vi "Drive Controller.vi"(8 "error in":errorcluster) -> ()   [LabVIEW 2017]
doc: "This VI executes continuously carrying out the current operation and responding to updates or new operation requests. It will often contain the timing or control code that is difficult to place directly in TeleOp. This VI generally opens all sensors and motors and isolates the rest of the robot code from knowing implementation details of how the operations are carried out."
uses:
  <vilib>/Rock Robotics/WPI/Framework/Completion Status.ctl
  Drive Setpoints.ctl
  Drive Operations.ctl
  <vilib>/Rock Robotics/WPI/SafetyOutput/WPI_SafetyOutputConfigMenu.ctl
  <vilib>/Rock Robotics/SystemInterfaces/DIO/FPGA_DIOChannel.ctl
  <vilib>/Rock Robotics/SystemInterfaces/DIO/FPGA_DIOPWMChannel.ctl
  <vilib>/Rock Robotics/WPI/Counter/WPI_CounterDigitalInputToDigitalSource.vi
  Framework/Robot Global Data.vi
  <vilib>/Rock Robotics/WPI/ThirdParty/Phoenix-LabVIEW/Pigeon IMU/CTRE_PigeonIMU_Open_TalonSRX.vi
  <vilib>/Rock Robotics/Network Tables/NT Write Number.vi
  <vilib>/Rock Robotics/WPI/RobotDrive/WPI_RobotDriveOpen4MotorWithSPARK.vi
  Support Code/Global Constants.vi
  <vilib>/Rock Robotics/Network Tables/NT Write Numeric Array.vi
panel:
  in  "PID Turn":T1={"proportional gain (Kc)"=0.015, "integral time (Ti, min)"=0.0, "derivative time (Td, min)"=0.0}
  in  "Sensitivity":dbl=0.2 format="%#_13g"
  out "Encoders":cluster{"Distance":dbl, "Distance":dbl}(graph)
  out "Left Encoder":dbl=-1185.6884765625
  out "Right Encoder":dbl=-1185.6884765625
  out "gyro":dbl=106.72
  out "Gyro":dbl(graph)=85.48
  in  "Interactive Values":T2={"Operation"=enum."Auto Turn", "Left Setpoint"=0.0, "Right Setpoint"=0.0, "Duration"=0.0, "Distance"=0.0, "Target Angle"=90.0, "Speed"=0.0}
  in  "Buttons":cluster{"Execute Cmd":bool, "Abort Cmd":bool}
  out "Command Timing":cluster{"Start Time (ms)":u32, "Iterations":i32}={"Start Time (ms)"=2214017, "Iterations"=0}
  out "Status":T4
  out "Setpoints":T5(graph)
  out "Current\nCmd":string="Started at  17:19:58.001\nDefault: Reserve,  L 0.0, R 0.0, D 0.000000, Dist 0.0, A 0.0, S 0.000000"
  # "Interactive Command: You may fill in the settings for a command\nand schedule it with the Execute button. You can observe and abort\nany command while fine tuning the code for the controller."
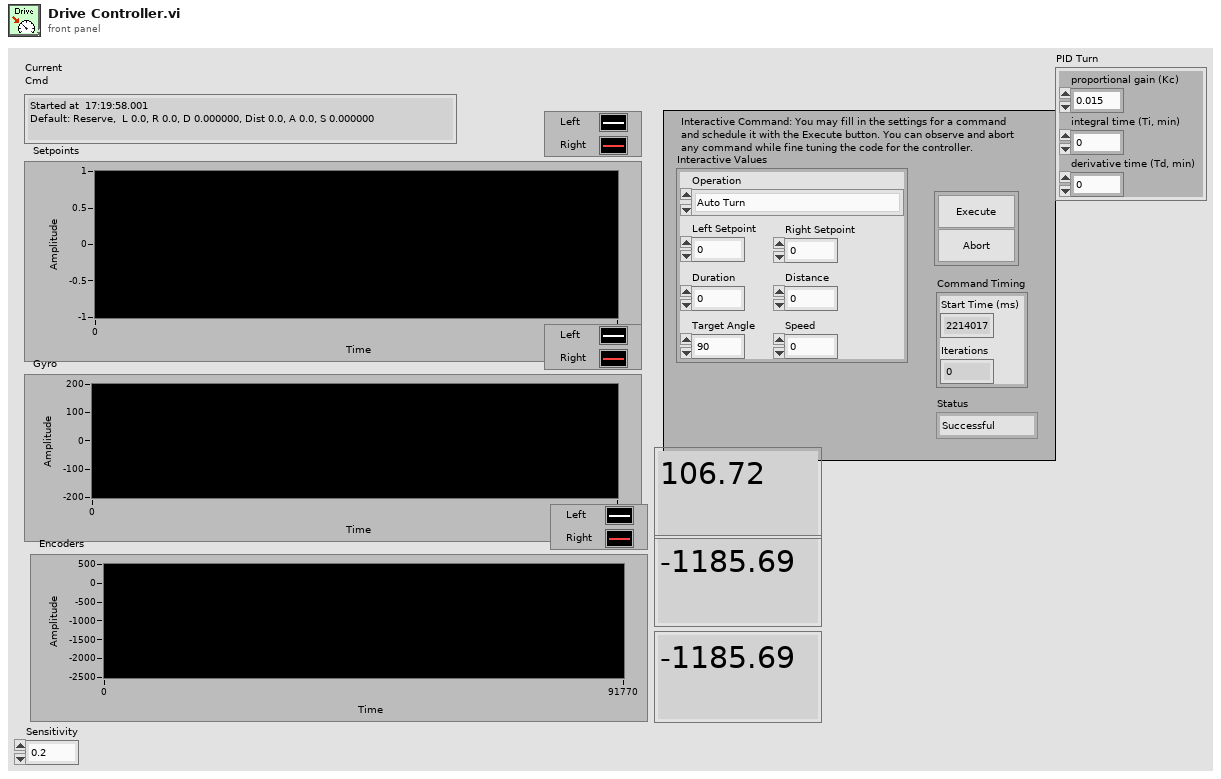
[diagram p1: front panel]
types:
  T1 = cluster{"proportional gain (Kc)":dbl, "integral time (Ti, min)":dbl, "derivative time (Td, min)":dbl}
  T2 = typedef "Drive Setpoints.ctl" = cluster{"Operation":T3, "Left Setpoint":dbl, "Right Setpoint":dbl, "Duration":dbl, "Distance":dbl, "Target Angle":dbl, "Speed":dbl}
  T3 = typedef "Drive Operations.ctl" = enum16{"Reserve", "Read Current", "Immediate", "Drive for Time", "Drive for Distance", "Drive PID", "Auto Turn", "Reset Encoders", "Reset Gyro"}
  T4 = typedef "Completion Status.ctl" = enum16{"Successful", "Aborted", "Incomplete"}
  T5 = cluster{"Left Setpoint":dbl, "Right Setpoint":dbl}
  T6 = typedef "FPGA_DIOPWMChannel.ctl" = enum8{"PWM 0", "PWM 1", "PWM 2", "PWM 3", "PWM 4", "PWM 5", "PWM 6", "PWM 7", "PWM 8", "PWM 9", "PWM MXP 0", "PWM MXP 1", "PWM MXP 2", "PWM MXP 3", "PWM MXP 4", "PWM MXP 5", "PWM MXP 6", "PWM MXP 7", "PWM MXP 8", "PWM MXP 9", "Invalid"}
  T7 = typedef "FPGA_DIOChannel.ctl" = enum8{"DIO 0", "DIO 1", "DIO 2", "DIO 3", "DIO 4", "DIO 5", "DIO 6", "DIO 7", "DIO 8", "DIO 9", "DIO MXP 0", "DIO MXP 1", "DIO MXP 2", "DIO MXP 3", "DIO MXP 4", "DIO MXP 5", "DIO MXP 6", "DIO MXP 7", "DIO MXP 8", "DIO MXP 9", "DIO MXP 10", "DIO MXP 11", "DIO MXP 12", "DIO MXP 13", "DIO MXP 14", "DIO MXP 15", "SPI Port CS1", "SPI Port CS2", "SPI Port CS3", "SPI Port MISO", "SPI Port MOSI", "Invalid"}
  T8 = typedef "WPI_SafetyOutputConfigMenu.ctl" = enum16{"Enable", "Disable"}
  T9 = typedef "WPI_MotorControlDeviceRef.ctl" = cluster{"DeviceStatus":errorcluster, "Type":T10, "PWM":cluster{"PWM Channel":T6, "DeadBand":T11}, "CAN":cluster{"Device Number":u8, "SetOutput VI Ref":variant, "GetOutput VI Ref":variant, "Enable VI Ref":variant, "Disable VI Ref":variant, "Data":variant}, "Invert":bool, "DIO PWM":cluster{"PWM \"Enable\" Channel":T6, "DIOChannel":T7, "PWM Rate":dbl}}
  T10 = typedef "WPI_MotorControlType.ctl" = enum16{"PWM", "CAN", "DIO PWM"}
  T11 = typedef "WPI_PWMDeadband.ctl" = cluster{"Name":string, "maxPositivePwm":i32, "minPositivePwm":i32, "centerPwm":i32, "maxNegativePwm":i32, "minNegativePwm":i32, "angularRange":u16}
  T12 = typedef "CTRE_PigeonIMU_DeviceRef.ctl" = cluster{"DeviceStatus":errorcluster, "Device Number":u8, "Type":T13, "Device ID":u32, "Handle":u64, "UsageFrame":u32, "Library Path":path}
  T13 = typedef "CTRE_PigeonIMU_ConnectionType.ctl" = u32
  T14 = typedef "WPI_DigitalInputDevRef.ctl" = cluster{"DevStatus":errorcluster, "DIO Channel":T7}
  T15 = typedef "WPI_RobotDriveDevRef.ctl" = cluster{"DevStatus":errorcluster, "Motors[]":T9[], "Square Inputs":bool, "Max Output":dbl}
  T16 = typedef "FPGA_CounterEncoderSourceConvertionLVSourceType.ctl" = cluster{"DevStatus":errorcluster, "AnalogTriggerMode?":bool, "DigitalMode":cluster{"DIO Channel":T17}, "AnalogTriggerMode":cluster{"AnalogTriggerIndex":T18, "OutputType":T19}}
  T17 = typedef "FPGA_DIODigitalSourceChannel.ctl" = enum8{"DIO 0", "DIO 1", "DIO 2", "DIO 3", "DIO 4", "DIO 5", "DIO 6", "DIO 7", "DIO 8", "DIO 9", "DIO MXP 0", "DIO MXP 1", "DIO MXP 2", "DIO MXP 3", "DIO MXP 4", "DIO MXP 5", "DIO MXP 6", "DIO MXP 7", "DIO MXP 8", "DIO MXP 9", "DIO MXP 10", "DIO MXP 11", "DIO MXP 12", "DIO MXP 13", "DIO MXP 14", "DIO MXP 15", "Disabled"}
  T18 = typedef "FPGA_AnalogTriggerIndex.ctl" = enum8{"Trig 0", "Trig 1", "Trig 2", "Trig 3", "Trig 4", "Trig 5", "Trig 6", "Trig 7", "Invalid"}
  T19 = typedef "FPGA_AnalogTriggerOutType.ctl" = enum16{"InWindow", "TriggerState", "Rising", "Falling"}
  T20 = typedef "WPI_EncoderDevRef.ctl" = cluster{"DevStatus":errorcluster, "EncoderIndex":T21, "CounterIndex":T22, "DistancePerCount":dbl, "Decoding Type":T23}
  T21 = typedef "FPGA_EncoderIdx.ctl" = enum8{"Enc 0", "Enc 1", "Enc 2", "Enc 3", "Enc 4", "Enc 5", "Enc 6", "Enc 7", "Invalid"}
  T22 = typedef "FPGA_CounterCtrSystemIndex.ctl" = enum8{"Ctr 0", "Ctr 1", "Ctr 2", "Ctr 3", "Ctr 4", "Ctr 5", "Ctr 6", "Ctr 7", "Invalid"}
  T23 = typedef "WPI_EncoderType.ctl" = enum16{"1x", "2x", "4x"}
  T24 = typedef "Command Status Info.ctl" = cluster{"Name":string, "Status":T4, "notifier out":T25}
  T25 = typedef "Completion Notifier.ctl" = refnum<notifier>
  T26 = cluster{"SubSystem Data":T2, cluster{"Start Time (ms)":u32, "Iterations":i32}, cluster{"Command Info":T24, "Description":string, "Default Command":T2, "queue out":refnum<queue>, "Subsystem Name":string}}
  T27 = cluster{"SubSystem Data":T2, cluster{"Start Time (ms)":u32, "Iterations":i32}, "Default Command Arguments":cluster{"Command Info":T24, "Description":string, "Default Command":T2, "queue out":refnum<queue>, "Subsystem Name":string}}
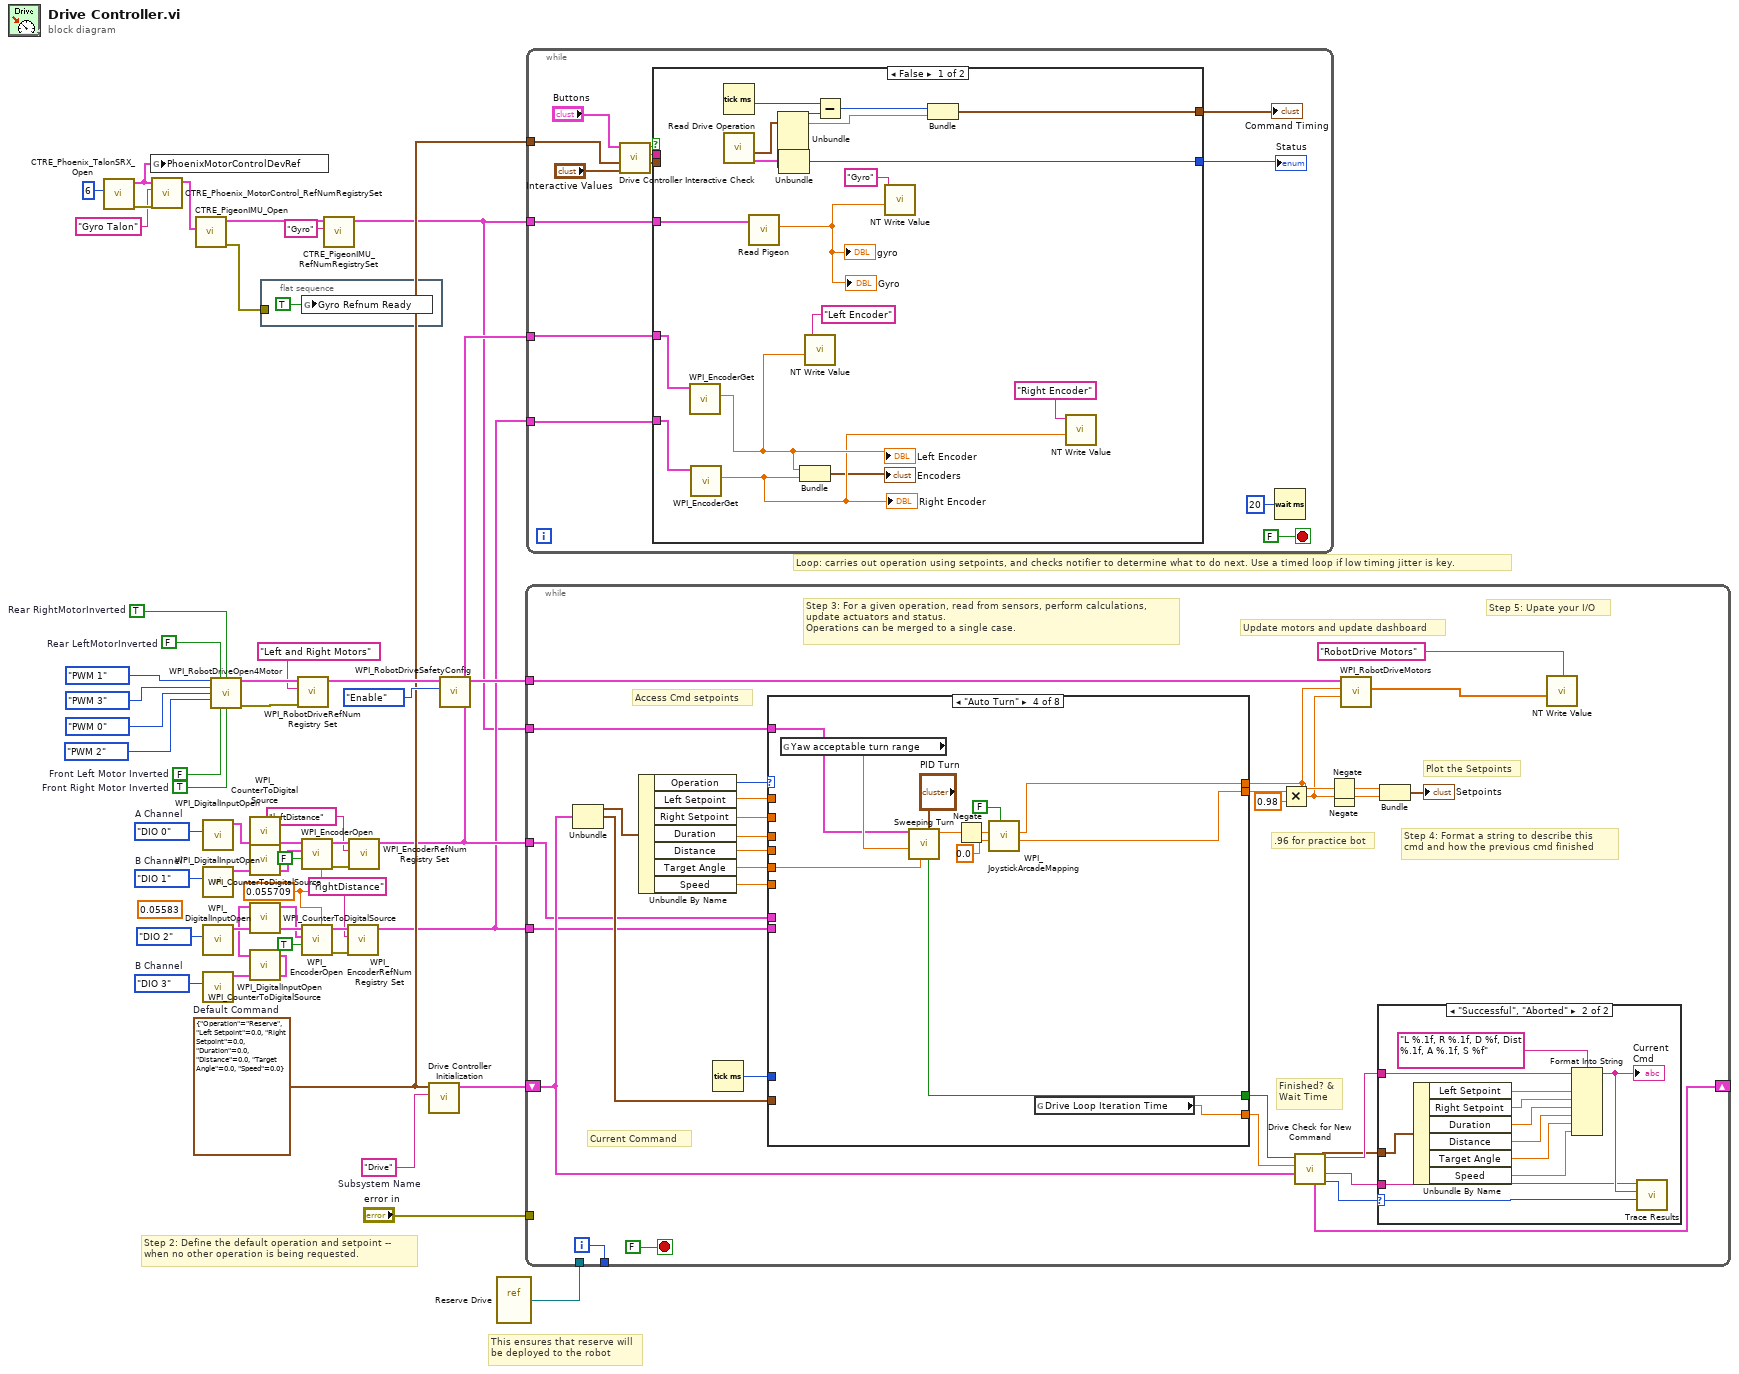
[diagram p0: block diagram]
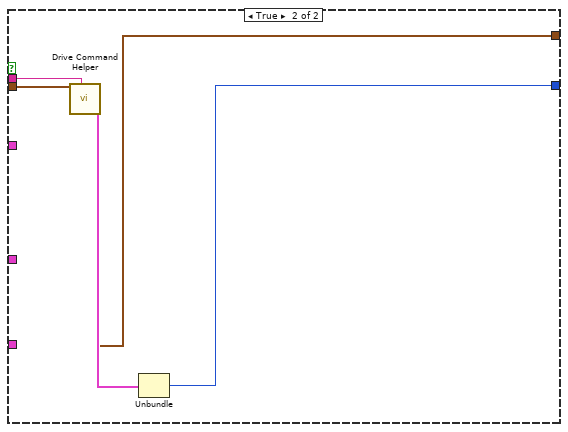
[diagram p2: hidden frame]
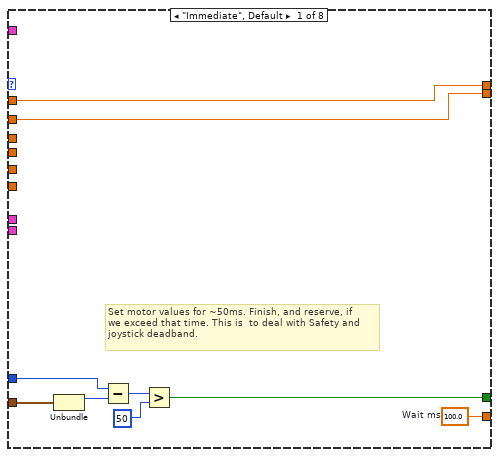
[diagram p4: hidden frame]
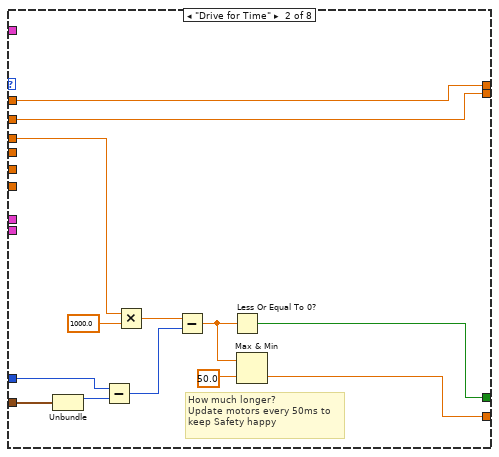
[diagram p5: hidden frame]
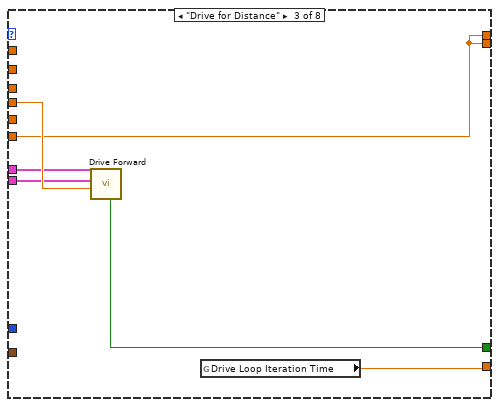
[diagram p6: hidden frame]
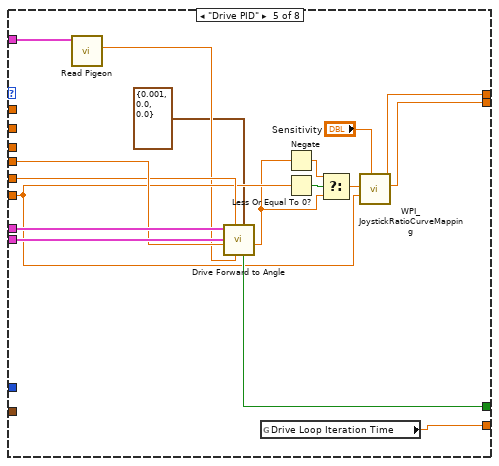
[diagram p7: hidden frame]
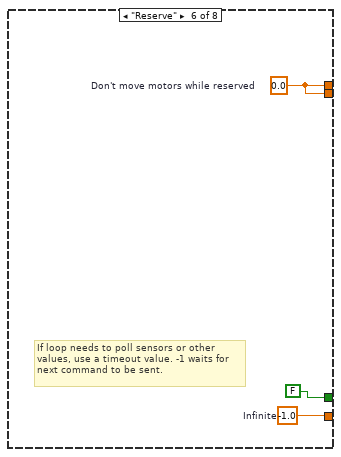
[diagram p8: hidden frame]
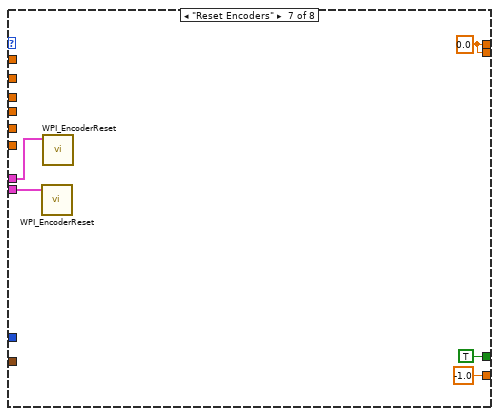
[diagram p9: hidden frame]
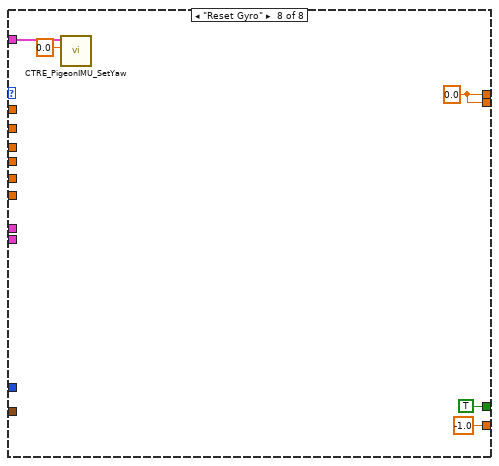
[diagram p10: hidden frame]
diagram:
  w2 = TRUE  # Front Right Motor Inverted
  w3 = FALSE  # Front Left Motor Inverted
  w8 = FALSE  # Rear LeftMotorInverted
  w9 = TRUE  # Rear RightMotorInverted
  w10 = 0.055709
  (unwired) 0.05583
  w31 = FPGA_DIOChannel."DIO 3"  # B Channel
  w40 = FPGA_DIOChannel."DIO 1"  # B Channel
  w39 = FPGA_DIOChannel."DIO 0"  # A Channel
  w41 = T2 {"Operation"=enum."Reserve", "Left Setpoint"=0.0, "Right Setpoint"=0.0, "Duration"=0.0, "Distance"=0.0, "Target Angle"=0.0, "Speed"=0.0}  # Default Command
  w51 = "Drive"  # Subsystem Name
  # "This ensures that reserve will\nbe deployed to the robot"
  # "Step 2: Define the default operation and setpoint --\nwhen no other operation is being requested."
  # "Loop: carries out operation using setpoints, and checks notifier to determine what to do next. Use a timed loop if low timing jitter is key."
  n1 = call <vilib>:"CTRE_Phoenix_TalonSRX_Open.vi"("Device Number"=u8 6) -> ("error out"=w17:errorcluster, "CAN Talon SRX Ref"=w1:T9)  [unwired: 9 in]
  n2 = global write "Robot Global Data.vi" "PhoenixMotorControlDevRef"(w1) -> ()
  n3 = call <vilib>:"CTRE_Phoenix_MotorControl_RefNumRegistrySet.vi"("error in (no error)"=w17, "refnum name"="Gyro Talon", "PhoenixMotorControlDevRef"=w1) -> ("PhoenixMotorControlDevRef"=w15:T9)  [unwired: 7 in, 1 out]
  n4 = call-poly <vilib>:"CTRE_PigeonIMU_Open.vi"("CAN Talon SRX Ref"=w15) -> ("error out"=w14:errorcluster, "PigeonIMUDevRef"=w13:T12)  [unwired: 9 in]
  n5 = call <vilib>:"WPI_DigitalInputOpen.vi"("DIO Channel"=w39) -> ("DigitalInputDevRef"=w36:T14)  [unwired: 1 in, 9 out]
  n6 = call <vilib>:"WPI_DigitalInputOpen.vi"("DIO Channel"=w40) -> ("DigitalInputDevRef"=w37:T14)  [unwired: 1 in, 9 out]
  n7 = call <vilib>:"WPI_DigitalInputOpen.vi"("DIO Channel"=FPGA_DIOChannel."DIO 2") -> ("DigitalInputDevRef"=w25:T14)  [unwired: 1 in, 9 out]
  n8 = call <vilib>:"WPI_DigitalInputOpen.vi"("DIO Channel"=w31) -> ("DigitalInputDevRef"=w30:T14)  [unwired: 1 in, 9 out]
  n9 = call-poly <vilib>:"WPI_RobotDriveOpen4Motor.vi"("Rear Left Motor"=FPGA_DIOPWMChannel."PWM 1", "Rear Left Motor Inverted"=w8, "Rear Right Motor Inverted"=w9, "Rear Right Motor"=FPGA_DIOPWMChannel."PWM 3", "Front Left Motor"=FPGA_DIOPWMChannel."PWM 0", "Front Right Motor"=FPGA_DIOPWMChannel."PWM 2", "Front Left Motor Inverted"=w3, "Front Right Motor Inverted"=w2) -> ("RobotDriveDevRef"=w50:T15, "error out"=w48:errorcluster)  [unwired: 6 in]
  n10 = call-poly <vilib>:"WPI_CounterToDigitalSource.vi"("DigitalInputDevRef"=w36) -> ("Digital Source"=w35:T16)  [unwired: 6 out]
  n11 = call-poly <vilib>:"WPI_CounterToDigitalSource.vi"("DigitalInputDevRef"=w37) -> ("Digital Source"=w38:T16)  [unwired: 6 out]
  n12 = call-poly <vilib>:"WPI_CounterToDigitalSource.vi"("DigitalInputDevRef"=w25) -> ("Digital Source"=w24:T16)  [unwired: 6 out]
  n13 = call-poly <vilib>:"WPI_CounterToDigitalSource.vi"("DigitalInputDevRef"=w30) -> ("Digital Source"=w23:T16)  [unwired: 6 out]
  n14 = flat-sequence {
    tunnel: w14 -> [_]
    frame #0 {
      n15 = global write "Robot Global Data.vi" "Gyro Refnum Ready"(TRUE ("Enable Vision")) -> ()
    }
  }
  n16 = call <vilib>:"WPI_RobotDriveRefNum Registry Set.vi"("error in (no error)"=w48, "refnum name"="Left and Right Motors", "RobotDriveDevRef"=w50) -> ("RobotDriveDevRef"=w47:T15)  [unwired: 1 in, 7 out]
  n17 = call <vilib>:"WPI_EncoderOpen.vi"("DistancePerCount"=w10, "Invert Direction (False)"=FALSE, "BSource"=w38, "ASource"=w35) -> ("error out"=w34:errorcluster, "EncoderDevRef"=w33:T20)  [unwired: 4 in, 2 out]
  n18 = call <vilib>:"WPI_EncoderOpen.vi"("DistancePerCount"=w10, "Invert Direction (False)"=TRUE, "BSource"=w23, "ASource"=w24) -> ("error out"=w29:errorcluster, "EncoderDevRef"=w28:T20)  [unwired: 4 in, 2 out]
  n19 = call <vilib>:"CTRE_PigeonIMU_RefNumRegistrySet.vi"("refnum name"="Gyro", "PigeonIMUDevRef"=w13) -> ("PigeonIMUDevRef"=w12:T12)  [unwired: 8 in, 1 out]
  n20 = call <vilib>:"WPI_EncoderRefNum Registry Set.vi"("error in (no error)"=w29, "refnum name"="rightDistance", "EncoderDevRef"=w28) -> ("EncoderDevRef"=w19:T20)  [unwired: 7 in, 1 out]
  n21 = call <vilib>:"WPI_EncoderRefNum Registry Set.vi"("error in (no error)"=w34, "refnum name"="leftDistance", "EncoderDevRef"=w33) -> ("EncoderDevRef"=w20:T20)  [unwired: 7 in, 1 out]
  n22 = call "Drive Controller Initialization.vi"("Subsystem Name"=w51, "Default Command"=w41) -> ("Current Command"=w43:T26)  [unwired: 9 in]
  n23 = call <vilib>:"WPI_RobotDriveSafetyConfig.vi"("mode"=WPI_SafetyOutputConfigMenu."Enable", "RobotDriveDevRef"=w47) -> ("RobotDriveDevRef"=w45:T15)  [unwired: 8 in, 1 out]
  n24 = vi-ref "Reserve Drive.vi"() -> (w42:refnum<vi>)
  n25 = while {
    shift-right: [w73] -> _
    shift-left: w43 -> [w66]
    tunnel: [w84] -> _
    tunnel: w45 -> [w81]
    tunnel: "error in" -> [_]
    tunnel: w42 -> [_]
    tunnel: w20 -> [w61]
    tunnel: w19 -> [w62]
    tunnel: w12 -> [w56]
    i -> [w84]
    stop <- FALSE stop-if-true
    # ".96 for practice bot"
    # "Step 5: Upate your I/O"
    # "Step 4: Format a string to describe this\ncmd and how the previous cmd finished"
    # "Current Command"
    # "Update motors and update dashboard"
    # "Plot the Setpoints"
    # "Access Cmd setpoints"
    # "Finished? &\nWait Time"
    # "Step 3: For a given operation, read from sensors, perform calculations,\nupdate actuators and status.\nOperations can be merged to a single case."
    n26 = Unbundle(w66) -> ("SubSystem Data"=w80:T2, w67:cluster{"Start Time (ms)":u32, "Iterations":i32})  [unwired: 1 out]
    n27 = Unbundle By Name(w80) -> ("Operation"=w79:T3, "Left Setpoint"=w78:dbl, "Right Setpoint"=w77:dbl, "Duration"=w76:dbl, "Distance"=w64:dbl, "Target Angle"=w63:dbl, "Speed"=w55:dbl)
    n28 = Tick Count (ms)() -> (millisecond timer value=w75:u32)
    n29 = case shown="\"Auto Turn\"" w79 {
      tunnel: [w106 w107 w120 w137 w147 w157 -1.0 ("Infinite") -1.0 ("Infinite")] -> w72
      tunnel: [w99 w114 w122 w136 w150 FALSE ("ignore previous (F)") TRUE ("ignore previous (F)") TRUE ("ignore previous (F)")] -> w71
      tunnel: w67 -> [w98 w116 _ _ _ _ _ _]
      tunnel: [w105 w113 w121 w132 w149 w155 w162 w167] -> w60
      tunnel: [w104 w112 w121 w131 w148 w155 w162 w167] -> w82
      tunnel: w78 -> [w105 w113 _ _ _ _ _ _]
      tunnel: w77 -> [w104 w112 _ _ _ _ _ _]
      tunnel: w76 -> [_ w111 _ _ _ _ _ _]
      tunnel: w75 -> [w100 w110 _ _ _ _ _ _]
      tunnel: w64 -> [_ _ w125 _ w152 _ _ _]
      tunnel: w63 -> [_ _ _ w130 w151 _ _ _]
      tunnel: w55 -> [_ _ w121 _ w146 _ _ _]
      tunnel: w62 -> [_ _ w124 _ w153 _ w159 _]
      tunnel: w61 -> [_ _ w123 _ w154 _ w158 _]
      tunnel: w56 -> [_ _ _ w127 w143 _ _ w164]
      frame "Immediate", Default {
        w106 = 100.0  # Wait ms
        # "Set motor values for ~50ms. Finish, and reserve, if\nwe exceed that time. This is  to deal with Safety and\njoystick deadband."
        n30 = Unbundle(w98) -> ("Start Time (ms)"=w101:u32)  [unwired: 1 out]
        n31 = Subtract(x=w100, y=w101) -> (x-y=w102:u32)
        n32 = Greater?(x=w102, y=u8 50 ("Left Motor")) -> (0:w99:bool)
      }
      frame "Drive for Time" {
        # "How much longer?\nUpdate motors every 50ms to\nkeep Safety happy"
        n33 = Unbundle(w116) -> ("Start Time (ms)"=w115:u32)  [unwired: 1 out]
        n34 = Subtract(x=w110, y=w115) -> (x-y=w119:u32)
        n35 = Multiply(x=w111, y=1000.0) -> (x*y=w118:dbl)
        n36 = Subtract(x=w118, y=w119) -> (x-y=w109:dbl)
        n37 = Less Or Equal To 0?(x=w109) -> (x <= 0?=w114:bool)
        n38 = Max & Min(x=w109, y=50.0) -> (min(x,y)=w107:dbl)  [unwired: 1 out]
      }
      frame "Drive for Distance" {
        n39 = call "Drive Forward.vi"("Distance"=w125, "rightDistance"=w124, "leftDistance"=w123) -> ("Stop"=w122:bool)  [unwired: 5 in, 3 out]
        n40 = global read "Global Constants.vi" "Drive Loop Iteration Time"() -> (w120:dbl)
      }
      frame "Auto Turn" {
        n41 = global read "Global Constants.vi" "Yaw acceptable turn range"() -> (w135:dbl)
        n42 = call "Sweeping Turn.vi"("PID gains"="PID Turn", "Target Yaw"=w130, "Acceptable Range"=w135, "PigeonIMUDevRef"=w127) -> ("Yaw Output"=w134:dbl, "Stop"=w136:bool)  [unwired: 4 in, 2 out]
        n43 = Negate(x=w134) -> (-x=w126:dbl)
        n44 = call <vilib>:"WPI_JoystickArcadeMapping.vi"("Square Inputs"=FALSE, "Y axis value"=0.0 ("Y axis value (Speed)"), "X axis value"=w126) -> ("Right Motor Value"=w131:dbl, "Left Motor Value"=w132:dbl)  [unwired: 7 in]
        n45 = global read "Global Constants.vi" "Drive Loop Iteration Time"() -> (w137:dbl)
      }
      frame "Drive PID" {
        n46 = call "Read Pigeon.vi"("PigeonIMUDevRef"=w143) -> ("Yaw"=w142:dbl)  [unwired: 10 in]
        n47 = call "Drive Forward to Angle.vi"("PID gains"=T1 {"proportional gain (Kc)"=0.001, "integral time (Ti, min)"=0.0, "derivative time (Td, min)"=0.0}, "yaw"=w142, "yaw setpoint"=w151, "Distance"=w152, "rightDistance"=w153, "leftDistance"=w154) -> ("yaw output"=w139:dbl, "Stop"=w150:bool)  [unwired: 1 in, 3 out]
        n48 = global read "Global Constants.vi" "Drive Loop Iteration Time"() -> (w147:dbl)
        n49 = Negate(x=w139) -> (-x=w138:dbl)
        n50 = Less Or Equal To 0?(x=w146) -> (x <= 0?=w145:bool)
        n51 = Select(t=w138, s=w145, f=w139) -> (s? t:f=w144:dbl)
        n52 = call <vilib>:"WPI_JoystickRatioCurveMapping.vi"("Sensitivity"="Sensitivity", "Y axis value (Speed)"=w146, "X axis value (Curve)"=w144) -> ("Right Motor Value"=w148:dbl, "Left Motor Value"=w149:dbl)  [unwired: 7 in]
      }
      frame "Reserve" {
        w155 = 0.0  # Don't move motors while reserved
        w157 = -1.0  # Infinite
        # "If loop needs to poll sensors or other\nvalues, use a timeout value. -1 waits for\nnext command to be sent."
      }
      frame "Reset Encoders" {
        w162 = 0.0 ("Don't move motors while reserved")
        n53 = call <vilib>:"WPI_EncoderReset.vi"("EncoderDevRef"=w159) -> ()  [unwired: 9 in, 2 out]
        n54 = call <vilib>:"WPI_EncoderReset.vi"("EncoderDevRef"=w158) -> ()  [unwired: 9 in, 2 out]
      }
      frame "Reset Gyro" {
        w167 = 0.0 ("Don't move motors while reserved")
        n55 = call <vilib>:"CTRE_PigeonIMU_SetYaw.vi"("Value"=0.0, "PigeonIMUDevRef"=w164) -> ()  [unwired: 8 in, 2 out]
      }
    }
    n56 = Multiply(x=w82, y=0.98) -> (x*y=w59:dbl)
    n57 = call "Drive Check for New Command.vi"("input cluster"=w66, "Wait time (ms)"=w72, "Finished?"=w71) -> ("Completion"=w74:T4, "Subsystem Name"=w68:string, "Current Command"=w69:T2, "Initial Trace String"=w70:string, "Next Command"=w73:T27)  [unwired: 4 in]
    n58 = Negate(x=w60) -> (-x=w58:dbl)
    n59 = Negate(x=w59) -> (-x=w57:dbl)
    n60 = call <vilib>:"WPI_RobotDriveMotors.vi"("RightSpeed"=w59, "LeftSpeed"=w60, "RobotDriveDevRef"=w81) -> ("Motor Values"=w53:dbl[])  [unwired: 1 in, 7 out]
    n61 = case shown="\"Successful\", \"Aborted\"" w74 {
      selector: w74 -> [_ w97]
      tunnel: w70 -> [_ w92]
      tunnel: w69 -> [_ w93]
      tunnel: w68 -> [_ w89]
      frame "Incomplete", Default {
        # "Continuing current command"
      }
      frame "Successful", "Aborted" {
        # "Report and setup for next command"
        n62 = Unbundle By Name(w93) -> ("Left Setpoint"=w95:dbl, "Right Setpoint"=w96:dbl, "Duration"=w90:dbl, "Distance"=w88:dbl, "Target Angle"=w87:dbl, "Speed"=w86:dbl)
        n63 = Format Into String(format string="L %.1f, R %.1f, D %f, Dist %.1f, A %.1f, S %f", initial string=w92, w95, w96, w90, w88, w87, w86) -> (resulting string=w91:string)  [unwired: 1 in, 1 out]
        "Current\nCmd" <- w91
        n64 = call <vilib>:"Trace Results.vi"("Status of previous command"=w97, "Description"=w91, "Subsystem"=w89) -> ()  [unwired: 9 in]
      }
    }
    n65 = Bundle(w58, w57) -> (→"Setpoints":cluster{dbl, dbl})  [unwired: 1 in]
    n66 = call-poly <vilib>:"NT Write Value.vi"("Numeric Array"=w53, "Name"="RobotDrive Motors") -> ()  [unwired: 9 in, 1 out]
  }
  n67 = while {
    tunnel: w41 -> [w172]
    tunnel: w12 -> [w170]
    tunnel: w20 -> [w169]
    tunnel: w19 -> [w168]
    stop <- FALSE stop-if-true
    n68 = call "Drive Controller Interactive Check.vi"("Interactive Command In"="Interactive Values", "Default Command"=w172, "Buttons"="Buttons") -> ("Interactive Command Out"=w174:T2, "Trace String"=w175:string, "Schedule"=w176:bool)  [unwired: 6 in]
    n69 = case shown="False" w176 {
      tunnel: [w195 w203] -> w177
      tunnel: [w194 w199] -> w178
      tunnel: w175 -> [_ w201]
      tunnel: w174 -> [_ w200]
      tunnel: w170 -> [w185 _]
      tunnel: w169 -> [w190 _]
      tunnel: w168 -> [w189 _]
      frame False {
        n70 = call <vilib>:"WPI_EncoderGet.vi"("EncoderDevRef"=w190) -> ("Distance"=w183:dbl)  [unwired: 5 in, 5 out]
        "Left Encoder" <- w183
        n71 = call <vilib>:"WPI_EncoderGet.vi"("EncoderDevRef"=w189) -> ("Distance"=w182:dbl)  [unwired: 5 in, 5 out]
        "Right Encoder" <- w182
        n72 = Tick Count (ms)() -> (millisecond timer value=w198:u32)
        n73 = call "Read Drive Operation.vi"() -> ("Command Info"=w192:T24, "SubSystem Data"=w191:T2)  [unwired: 9 in, 1 out]
        n74 = call "Read Pigeon.vi"("PigeonIMUDevRef"=w185) -> ("Yaw"=w184:dbl)  [unwired: 10 in]
        "gyro" <- w184
        "Gyro" <- w184
        n75 = Unbundle(w191) -> ("Operation"=w196:T3, "Left Setpoint"=w193:dbl)  [unwired: 5 out]
        n76 = Unbundle(w192) -> ("Status"=w195:T4)  [unwired: 2 out]
        n77 = Bundle("Distance"=w183, "Distance"=w182) -> (→"Encoders":cluster{"Distance":dbl, "Distance":dbl})  [unwired: 1 in]
        n78 = call-poly <vilib>:"NT Write Value.vi"("Numeric"=w183, "Name"="Left Encoder") -> ()  [unwired: 9 in, 1 out]
        n79 = Subtract(x=w198, y=w196) -> (x-y=w197:u32)
        n80 = call-poly <vilib>:"NT Write Value.vi"("Numeric"=w184, "Name"="Gyro") -> ()  [unwired: 9 in, 1 out]
        n81 = Bundle(w197, "Left Setpoint"=w193) -> (w194:cluster{u32, "Left Setpoint":dbl})  [unwired: 1 in]
        n82 = call-poly <vilib>:"NT Write Value.vi"("Numeric"=w182, "Name"="Right Encoder") -> ()  [unwired: 9 in, 1 out]
      }
      frame True {
        n83 = call "Drive Command Helper.vi"("Description"=w201, "SubSystem Data"=w200) -> ("Command Info Out"=w202:T24, "Command Timing"=w199:cluster{"Start Time (ms)":u32, "Iterations":i32})  [unwired: 7 in, 1 out]
        n84 = Unbundle(w202) -> ("Status"=w203:T4)  [unwired: 2 out]
      }
    }
    "Status" <- w177
    "Command Timing" <- w178
    n85 = Wait (ms)(milliseconds to wait=u32 20) -> ()  [unwired: 1 out]
  }
